vi "Write Instruments.vi"(8 "error in (no error)":errorcluster, 10 "Instruments":T1, 11 "Control Experiment SM in":refnum<class "Control Experiment SM.lvclass">) -> (0 "error out":errorcluster, 3 "Control Experiment SM out":refnum<class "Control Experiment SM.lvclass">)   [LabVIEW 2016, in "Control Experiment SM.lvclass"]
uses:
  Control Experiment SM.lvclass
  Typedefs/Instruments--cluster.ctl
  <userlib>/LevyLab/Lockin-Multichannel/Instrument.Lockin/Instrument.Lockin.lvclass
  <userlib>/LevyLab/Levylab Instruments/Instrument Types/Cryostat/Instrument.Cryostat.lvclass
  <userlib>/LevyLab/Levylab Instruments/Instrument Types/CBridge/Instrument.CBridge.lvclass
  <userlib>/LevyLab/Levylab Instruments/Instrument Types/Optical Delay Line/Instrument.OpticalDelayLine.lvclass
  <userlib>/LevyLab/Levylab Instruments/Instrument Types/Strain/Instrument.Strain.lvclass
  <userlib>/LevyLab/Levylab Instruments/Instrument Types/VNA/Instrument.VNA.lvclass
  <userlib>/LevyLab/Levylab Instruments/Instrument Types/VSource/Instrument.VSource.lvclass
  <userlib>/LevyLab/Krohn Hite 7008/Instrument.KH7008.lvclass
  Control Experiment SM.lvclass/Control Experiment SM.ctl
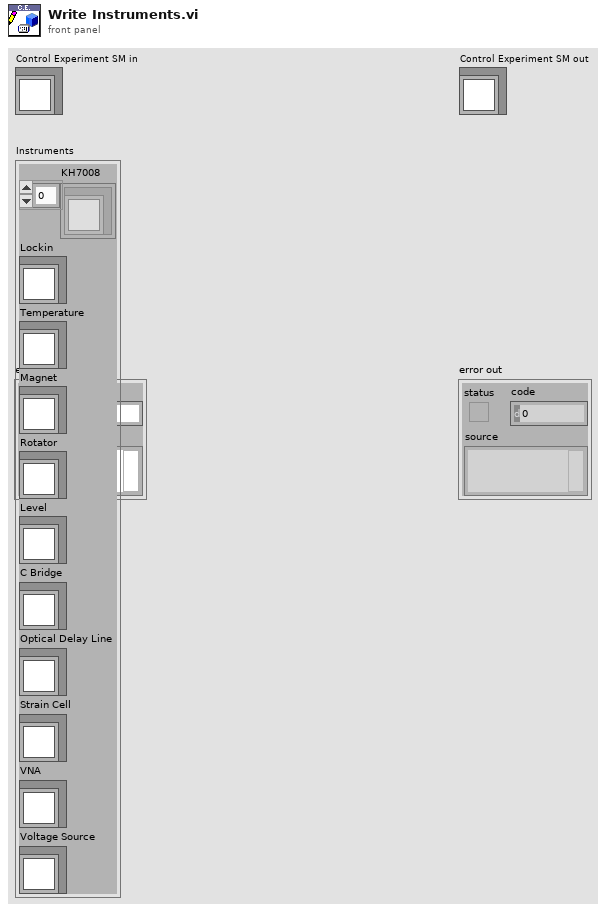
[diagram p1: front panel]
types:
  T1 = typedef "Control Experiment SM.lvclass/Instruments--cluster.ctl" = cluster{"KH7008":refnum<class "Instrument.KH7008.lvclass">[], "Lockin":refnum<class "Instrument.Lockin.lvclass">, "Temperature":refnum<class "Instrument.Cryostat.lvclass">, "Magnet":refnum<class "Instrument.Cryostat.lvclass">, "Rotator":refnum<class "Instrument.Cryostat.lvclass">, "Level":refnum<class "Instrument.Cryostat.lvclass">, "C Bridge":refnum<class "Instrument.CBridge.lvclass">, "Optical Delay Line":refnum<class "Instrument.OpticalDelayLine.lvclass">, "Strain Cell":refnum<class "Instrument.Strain.lvclass">, "VNA":refnum<class "Instrument.VNA.lvclass">, "Voltage Source":refnum<class "Instrument.VSource.lvclass">}
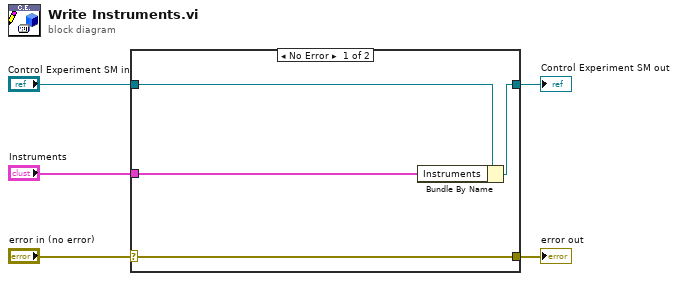
[diagram p0: block diagram]
diagram:
  n1 = case shown="No Error" "error in (no error)" {
    selector: "error in (no error)" -> [w9 w10]
    tunnel: [w9 w10] -> w4
    tunnel: [w7 w11] -> w2
    tunnel: "Control Experiment SM in" -> [w8 w11]
    tunnel: "Instruments" -> [w6 _]
    frame No Error {
      n2 = Bundle By Name(cluster=w8, "Instruments"=w6) -> (w7:refnum<class "Control Experiment SM.lvclass">)
    }
    frame Error {
    }
  }
  "error out" <- w4
  "Control Experiment SM out" <- w2
